vi "Write SEQ Frame.vi"(4 "error in (no error)":errorcluster, 5 "Image In":T1, 6 "AOI List":u16[][](array[numeric]), 7 "Seq file refnum":refnum<file>) -> (0 "error out":errorcluster, 3 "dup refnum":refnum<file>)   [LabVIEW 2016]
doc: "Write SEQ Frame.vi\n\nThe VI converts one frame of the 2D U8 array of pixels to the SEQ compressed format. This VI follows faithfully the compression function for a line (compress) in c:\\msdev\\convert.cpp (and the for loop to account for the entire frame). What has been added is the two exterior for loops of the VI, which effectively \"cut out\" the AOIs to convert and save, disregarding the rest of the frame.\n\nTo understand this code, it's important to have a copy of the C++ code in front of you. Rather than describe step by step what is happening, I'll explain the logistics of the program. I'll start within the second for loop (loop each aoi col). Only two params are passed into this loop, the 2D array of pixels (for one frame with a single AOI specified) and the length of the AOI row. The frame is separated into individual lines immediately. It's important to note that compression is done on a line to line basis, so nothing needs to be passed from column to column, although cumulative information about the frame as a whole is stored in the first two pixels of the SEQ file.\n A *result array is created near the array indexing. This is where the compressed line of the SEQ image will be saved. It is 1024 long even though the max line length is 512. Why is that? Because of the nature of the compression function, the size of the file can actually increase if there is a checkered effect along the line (bright white pixel, dark black pixel, bright white...etc.) This is because the compression function saves room only when there are small variations in brightness and actually takes up more room when the brightness changes often.\n The first pixel of the line is stored as the third element of the *result array. (The first two will be filled at the end). The line array is then passed to something called s. This is slightly tricky. The program constantly needs the information of the current pixel and the previous pixel to do the compression. The array wire marked pixel array is the last pixel while the s array is the current. I make the s array always one element ahead of the pixel array by pushing the first element of the array to the last position and moving everything up one, so the first element of s is the second element of pixel array, and so on. There are also a few other variables here such as d, d nibble, and low which I will describe later.\n Now, let's consider the actual compression function. This is the inner for loop. It's easier to visualize what's going on if you look at the C++ code. This for loop mimmicks the while loop in the C++ code. The small case box on the left upper corner of the for loop stands for the if/else part of the code. This case structure finds the absolute value difference between the pixel and s pixels (old and new).\n The larger case structure to the right of this one contains the meat of the program. The outer T/F question is whether the difference between pixels is greater than seven or less than -7. This number difference is the actual variation of brightness between the two pixels. If it's too large of a difference (as in the true case), then we're out of luck and we need to store the new pixel.\n There is a further complication to the matter, and that is which nibble we're saving into. The nibble is half of a pixel, and this can change when we actually do compression and don't use a full byte of storage for the pixel's information. There is a case loop within the true case, and this depends on the the nibble state which is either high or low. I use a boolean statement to represent this, with true meaning low and false meaning high. If we are on the high nibble the pixel is easier to save, so let's look at the false case first.\n Here you'll notice d multiple times. the d nibble is passed in and added to the binary code marked *d, and another integer simply called d is passed in and incremented twice. In the C++ code, this takes up two lines. The first adds (bitwise) the d nibble to the flag F0 and the second stores the full pixel in the result buffer. This occurs in the VI, but with some added things.\n First of all, the d nibble is a variable that is shift registered through this inner for loop. The *d flag, F0, never changes. This is a marker for the SEQ reading program that the pixel difference overflowed so a new pixel will immediately follow the flag. This case is only possible if the file is on a high nibble, so the low nibble will be actual data. However, this data has not yet been saved in my version of the program, instead it has been passed in from the previous looping as the d nibble. When it is combined with the F0, the data is stored in the '0' half of the byte. To visualize what is happening, the 'F' is the high nibble and the '0' is the low nibble. The bitwise And combines them into a full byte, which I then write to the result array. But at which element of the array? This is the purpose of the d integer. D specifies where to save the byte. Then d is incremented and then s (the current pixel) is saved to the result array and d is incremented again. We reverse the nibble state to low and go into the loop again.\n Let us now consider the 'true' of that nibble state case structure. In the C++ code, the flag 0F is stored in the right hand nibble then the first half of the pixel is stored in the left hand nibble (by logically shifting 4 bits to the left) and finally the second half of the pixel is stored in the right hand nibble of the next byte. In the VI, I had to approach this differently. First, the current pixel, s, is passed in, shifted to the left, and Anded to the 0F flag. Then it is saved in the result array. D is incremented and then the second half of the pixel is shifted to the right and passed to the shift register. Unlike the code, the VI doesn't store the half-pixel immediately. If you go back to the false case, you can understand how on the following loop iteration, the d nibble will be ready to be stored. All of this is done so that only full bytes will be stored in the array rather than half bytes which would need to be extracted, amended, and replaced.\n Well, now you should understand how the program is running thus far, although no compression has actually been done yet! To see that, go to the outer case structure and go to false. This is similar to the true case in that it also has a low/high nibble case structure, but no pixels are stored here. There is also an if/else case, as in the code, to force the difference to be positive. In the nibble state case of low, the difference is stored as the d nibble and passed to the shift register. In the false case (high), the d nibble is Anded to the difference and stored in the result array, and d in incremented.\n Well, there it is. There are certain clean up procedures that follow each line compression, however. First, if the line ends on the high nibble, d is incremented. There is also a big fuss to save info and flags in the first two bytes of the line. I haven't even thought through exactly what or how this works; I just copied the C++ code (the bptr and bptr+1 data). I know it must save flag information for the SEQ reading program to differentiate lines and info on the length of each line."
uses:
  <vilib>/vision/Image Controls.llb/IMAQ Image.ctl
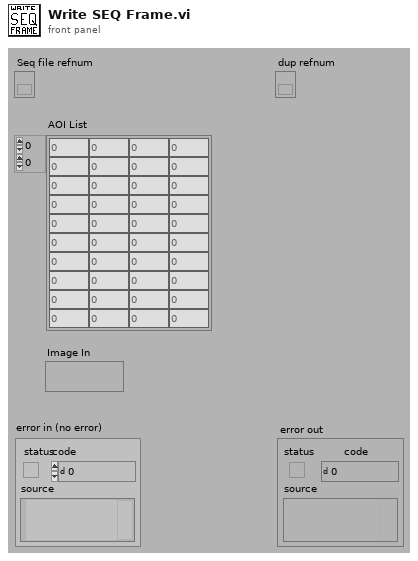
[diagram p1: front panel]
types:
  T1 = typedef "IMAQ Image.ctl" = refnum<image>
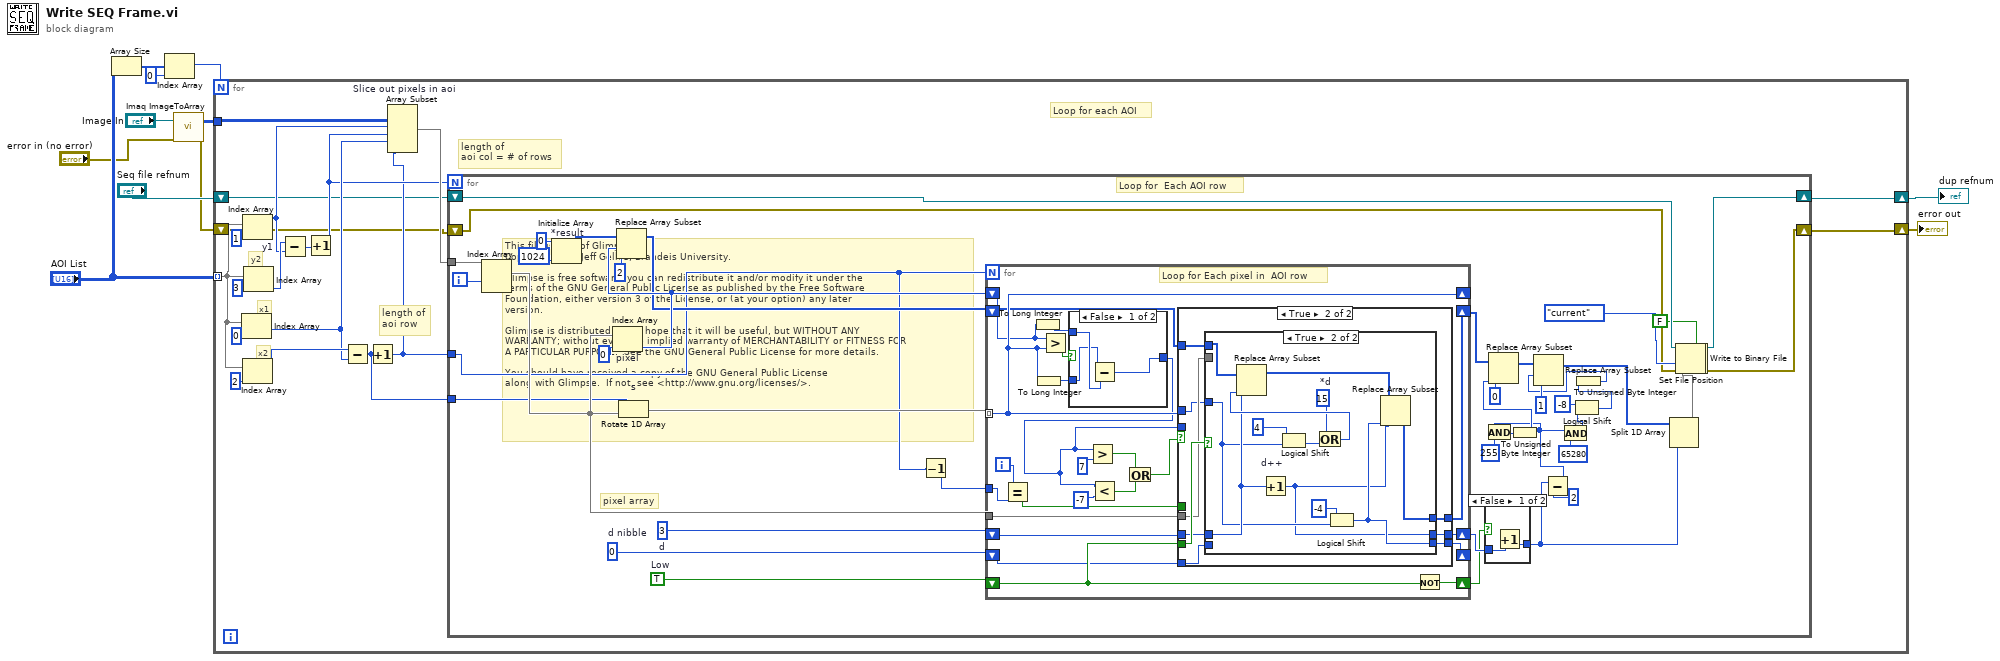
[diagram p0: block diagram]
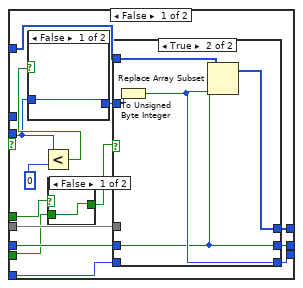
[diagram p3: hidden frame]
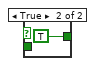
[diagram p4: hidden frame]
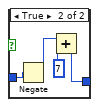
[diagram p5: hidden frame]
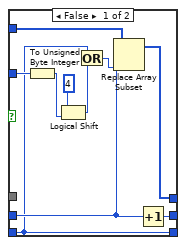
[diagram p6: hidden frame]
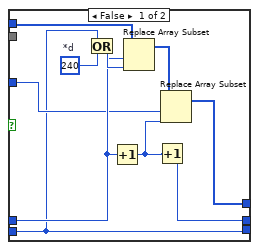
[diagram p7: hidden frame]
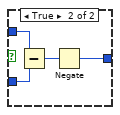
[diagram p8: hidden frame]
diagram:
  # "This file is part of Glimpse. \nCopyright 2014 Jeff Gelles, Brandeis University.    \n\nGlimpse is free software: you can redistribute it and/or modify it under the \nterms of the GNU General Public License as published by the Free Software \nFoundation, either version 3 of the License, or (at your option) any later \nversion.\n\nGlimpse is distributed in the hope that it will be useful, but WITHOUT ANY \nWARRANTY; without even the implied warranty of MERCHANTABILITY or FITNESS FOR \nA PARTICULAR PURPOSE.  See the GNU General Public License for more details.\n\nYou should have received a copy of the GNU General Public License\nalong with Glimpse.  If not, see <http://www.gnu.org/licenses/>."
  n1 = Array Size(array="AOI List") -> (size(s)=w10:i32[])
  n2 = Index Array(array=w10, index=0) -> (element=w9:i32)
  n3 = call "Imaq ImageToArray"("error in (no error)"="error in (no error)", "Image"="Image In") -> ("error out"=w2:errorcluster, "Image Pixels (U8)"=w8:u8[][])  [unwired: 1 in, 4 out]
  n4 = for {
    N: w9 -> [_]
    tunnel: w8 -> [w30]
    tunnel: "AOI List" -> [w24] mode=indexing
    shift-right: [w15] -> w5
    shift-left: "Seq file refnum" -> [w13]
    shift-right: [w14] -> w4
    shift-left: w2 -> [w12]
    # "x2"
    # "x1"
    # "y2"
    # "Loop for each AOI"
    # "length of\naoi col = # of rows"
    # "length of\naoi row"
    n5 = Index Array(array=w24, index=0) -> (element=w20:u16)
    n6 = Index Array "y1"(array=w24, index=1) -> (element=w22:u16)
    n7 = Index Array(array=w24, index=2) -> (element=w21:u16)
    n8 = Index Array(array=w24, index=3) -> (element=w23:u16)
    n9 = Subtract(x=w23, y=w22) -> (x-y=w19:u16)
    n10 = Increment(x=w19) -> (x+1=w18:u16)
    n11 = Subtract(x=w21, y=w20) -> (x-y=w17:u16)
    n12 = Increment(x=w17) -> (x+1=w16:u16)
    n13 = Array Subset "Slice out pixels in aoi"(array=w30, index (row)=w22, length (row)=w18, index (col)=w20, length (col)=w16) -> (w29:u8[][])
    n14 = for {
      N: w18 -> [_]
      tunnel: w29 -> [w74]
      tunnel: w16 -> [w39]
      tunnel: w17 -> [w38]
      shift-right: [w37] -> w15
      shift-left: w13 -> [w35]
      shift-right: [w36] -> w14
      shift-left: w12 -> [w34]
      i -> [w58]
      w54 = u8 0  # d nibble
      w70 = TRUE  # Low
      w71 = 3  # d
      # "Loop for  Each AOI row"
      # "pixel array"
      n15 = Index Array(array=w74, index (row)=w58) -> (element=w55:u8[])  [unwired: 1 in]
      n16 = Initialize Array "*result"(u8 0, 1024) -> (w57:u8[])
      n17 = Index Array "pixel"(array=w55, index=0) -> (element=w45:u8)
      n18 = Replace Array Subset(array=w57, new element=w45, index=2) -> (w43:u8[])
      n19 = Rotate 1D Array "s"(1:w55, 2:w38) -> (0:w72:u8[])
      n20 = Decrement(x=w39) -> (x-1=w41:u16)
      n21 = for {
        N: w39 -> [_]
        shift-right: [w89] -> _
        shift-left: w45 -> [w87]
        tunnel: w72 -> [w89] mode=indexing
        shift-right: [w94] -> w69
        shift-left: w71 -> [w91]
        shift-right: [w92] -> w40
        shift-left: w70 -> [w93]
        shift-right: [w85] -> w56
        shift-left: w43 -> [w86]
        tunnel: w55 -> [w84]
        shift-right: [w83] -> _
        shift-left: w54 -> [w82]
        tunnel: w41 -> [w80]
        i -> [w79]
        # "Loop for Each pixel in  AOI row"
        n22 = Equal?(x=w79, y=w80) -> (x = y?=w78:bool)
        n23 = To Long Integer ("difference")(number=w87) -> (32bit integer=w88:i32)
        n24 = To Long Integer ("difference")(number=w89) -> (32bit integer=w90:i32)
        n25 = Greater?(x=w87, y=w89) -> (0:w100:bool)
        n26 = case shown="False" w100 {
          tunnel: w88 -> [w170 w173]
          tunnel: w90 -> [w168 w174]
          tunnel: [w169 w171] -> w81
          frame False {
            n27 = Subtract(x=w168, y=w170) -> (x-y=w169:i32)
          }
          frame True {
            n28 = Subtract(x=w173, y=w174) -> (x-y=w172:i32)
            n29 = Negate(x=w172) -> (-x=w171:i32)
          }
        }
        n30 = Greater?(x=w81, y=7) -> (0:w98:bool)
        n31 = Less?(x=w81, y=-7) -> (x < y?=w96:bool)
        n32 = Or(x=w98, y=w96) -> (x .or. y?=w95:bool)
        n33 = case shown="True" w95 {
          tunnel: w93 -> [w102 w145]
          tunnel: w81 -> [w112 _]
          tunnel: w84 -> [w110 w144]
          tunnel: w89 -> [_ w143]
          tunnel: w91 -> [w109 w142]
          tunnel: [w107 w141] -> w94
          tunnel: [w108 w140] -> w85
          tunnel: w86 -> [w106 w139]
          tunnel: [w104 w138] -> w83
          tunnel: w82 -> [w105 w137]
          tunnel: w78 -> [w103 _]
          frame False {
            n34 = Less?(x=w112, y=0) -> (x < y?=w113:bool)
            n35 = case shown="False" w113 {
              tunnel: w112 -> [w117 w121]
              tunnel: [w117 w118] -> w111
              frame False {
              }
              frame True {
                n36 = Negate(x=w121) -> (-x=w120:i32)
                n37 = Add(x=w120, y=7) -> (x+y=w118:i32)
              }
            }
            n38 = case shown="False" w103 {
              tunnel: [w115 TRUE] -> w101
              tunnel: w102 -> [w115 _]
              frame False {
              }
              frame True {
              }
            }
            n39 = case shown="True" w101 {
              tunnel: w111 -> [w124 w136]
              tunnel: w110 -> [_ _]
              tunnel: w109 -> [w129 w132]
              tunnel: [w130 w134] -> w108
              tunnel: [w128 w132] -> w107
              tunnel: w106 -> [w127 w135]
              tunnel: w105 -> [w122 _]
              tunnel: [w122 w133] -> w104
              frame False {
                n40 = To Unsigned Byte Integer(number=w124) -> (unsigned 8bit integer=w125:u8)
                n41 = Logical Shift(y=i16 4, x=w125) -> (x << y=w123:u8)
                n42 = Or(x=w122, y=w123) -> (x .or. y?=w126:u8)
                n43 = Replace Array Subset(array=w127, new element=w126, index=w129) -> (w130:u8[])
                n44 = Increment(x=w129) -> (x+1=w128:i32)
              }
              frame True {
                n45 = To Unsigned Byte Integer(number=w136) -> (unsigned 8bit integer=w133:u8)
                n46 = Replace Array Subset(array=w135, new element=w133, index=w132) -> (w134:u8[])
              }
            }
          }
          frame True {
            n47 = case shown="True" w145 {
              tunnel: w144 -> [_ _]
              tunnel: w143 -> [w151 w162]
              tunnel: w142 -> [w152 w164]
              tunnel: [w149 w156] -> w141
              tunnel: [w148 w158] -> w140
              tunnel: w139 -> [w147 w161]
              tunnel: [w146 w157] -> w138
              tunnel: w137 -> [w146 _]
              frame False {
                w155 = u8 240  # *d
                n48 = Or(x=w146, y=w155) -> (x .or. y?=w154:u8)
                n49 = Increment(x=w152) -> (x+1=w150:i32)
                n50 = Replace Array Subset(array=w147, new element=w154, index=w152) -> (w153:u8[])
                n51 = Increment(x=w150) -> (x+1=w149:i32)
                n52 = Replace Array Subset(array=w153, new element=w151, index=w150) -> (w148:u8[])
              }
              frame True {
                w160 = u8 15  # *d
                n53 = Increment "d++"(x=w164) -> (x+1=w156:i32)
                n54 = Logical Shift(y=i16 4, x=w162) -> (x << y=w167:u8)
                n55 = Or(x=w160, y=w167) -> (x .or. y?=w165:u8)
                n56 = Replace Array Subset(array=w161, new element=w165, index=w164) -> (w159:u8[])
                n57 = Logical Shift(y=i8 -4 ("x"), x=w162) -> (x << y=w157:u8)
                n58 = Replace Array Subset(array=w159, new element=w157, index=w156) -> (w158:u8[])
              }
            }
          }
        }
        n59 = Not(x=w93) -> (.not. x?=w92:bool)
      }
      n60 = case shown="False" w40 {
        tunnel: w69 -> [w76 w77]
        tunnel: [w75 w77] -> w50
        frame False {
          n61 = Increment(x=w76) -> (x+1=w75:i32)
        }
        frame True {
        }
      }
      n62 = Subtract(x=w50, y=2 ("d")) -> (x-y=w49:i32)
      n63 = And(x=w49, y=u8 255) -> (x .and. y?=w60:i32)
      n64 = To Unsigned Byte Integer(number=w60) -> (unsigned 8bit integer=w59:u8)
      n65 = Replace Array Subset(array=w56, new element=w59, index=0) -> (w65:u8[])
      n66 = And(x=w49, y=u16 65280) -> (x .and. y?=w48:i32)
      n67 = Logical Shift(y=i16 -8, x=w48) -> (x << y=w47:i32)
      n68 = To Unsigned Byte Integer(number=w47) -> (unsigned 8bit integer=w46:u8)
      n69 = Replace Array Subset(array=w65, new element=w46, index=1) -> (w52:u8[])
      n70 = Split 1D Array(array=w52, index=w50) -> (first subarray=w42:u8[])  [unwired: 1 out]
      n71 = Set File Position(refnum=w35, from (0:start)=enum16{"start", "end", "current"}."current" ("pos mode (0:2)"), error in=w34) -> (refnum out=w33:refnum<file>, error out=w32:errorcluster)  [unwired: 1 out]
      n72 = Write to Binary File(file (use dialog)=w33, data=w42, error in=w32, 5:FALSE ("prepend array or string size? (T)")) -> (refnum out=w37:refnum<file>, error out=w36:errorcluster)  [unwired: 3 out]
    }
  }
  "dup refnum" <- w5
  "error out" <- w4
